vi "find_PrepLineObject_by_Koords.vi"(9 "Coords":T1, 10 "PrepLine\nobjects in":refnum<class "PrepLineObject.lvclass">[](array[class])) -> (0 "changed PrepLineObject":refnum<class "PrepLineObject.lvclass">, 1 "name of changed":string, 2 "changed switch array":bool[](array[boolean]), 3 "PrepLineObjectsOut":refnum<class "PrepLineObject.lvclass">[](array[class]))   [LabVIEW 2017]
doc: "According to coordinates the correct PrepLineObject is located by looking through the Array of all PrepLineObjects (stored in a queue). The output array has the same size as the array with the switch objects and shows (state = true) the location of the Object that that has been selected."
uses:
  <vilib>/Utility/miscctls.llb/LVPoint32TypeDef.ctl
  Classes/PrepLineObject/PrepLineObject.lvclass
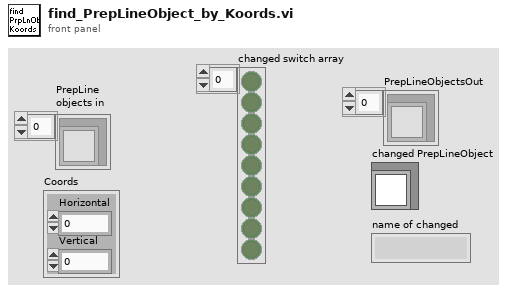
[diagram p1: front panel]
types:
  T1 = typedef "LVPoint32TypeDef.ctl" = cluster{"Horizontal":i32, "Vertical":i32}
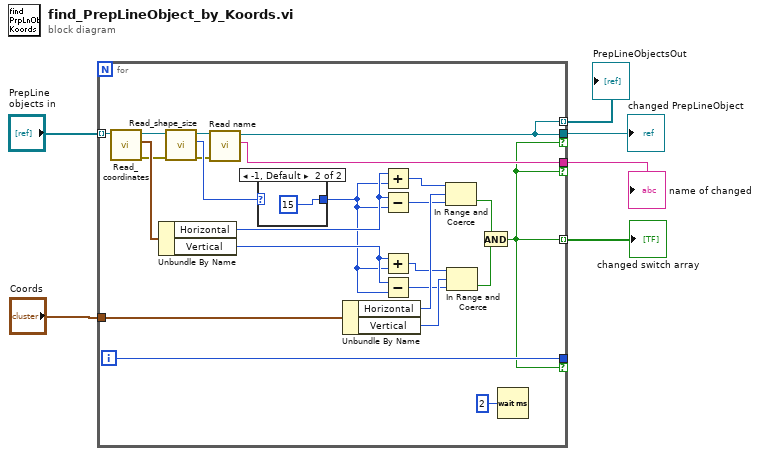
[diagram p0: block diagram]
diagram:
  n1 = for {
    tunnel: "PrepLine\nobjects in" -> [w30] mode=indexing
    tunnel: "Coords" -> [w28]
    tunnel: [w7] -> w5 mode=indexing
    tunnel: [w10] -> w4 if=w7
    tunnel: [w11] -> w3 if=w7
    tunnel: [w10] -> w1 mode=indexing
    tunnel: [w8] -> _ if=w7
    i -> [w8]
    n2 = call-dynamic "Read_coordinates.vi"("PrepLinePictureObjects in"=w30) -> ("PrepLinePictureObjects out"=w27:refnum<class "PrepLineObject.lvclass">, "Coords"=w29:T1, "error out"=w26:errorcluster)  [unwired: 7 in]
    n3 = Unbundle By Name(w29) -> ("Horizontal"=w24:i32, "Vertical"=w22:i32)
    n4 = call-dynamic "Read_shape_size.vi"("PrepLinePictureObjects in"=w27, "error in (no error)"=w26) -> ("PrepLinePictureObjects out"=w13:refnum<class "PrepLineObject.lvclass">, "shape type"=w15:i8, "error out"=w12:errorcluster)  [unwired: 6 in]
    n5 = call-dynamic "Read name.vi"("error in (no error)"=w12, "PrepLineObject in"=w13) -> ("name"=w11:string, "PrepLineObject out"=w10:refnum<class "PrepLineObject.lvclass">)  [unwired: 7 in, 1 out]
    n6 = case shown="-1, Default" w15 {
      selector: w15 -> [w31 _]
      tunnel: [w31 i8 15 ("shape type")] -> w14
      frame 0.. {
      }
      frame -1, Default {
      }
    }
    n7 = Unbundle By Name(w28) -> ("Horizontal"=w23:i32, "Vertical"=w25:i32)
    n8 = Add(x=w24, y=w14) -> (x+y=w21:i32)
    n9 = Subtract(x=w24, y=w14) -> (x-y=w20:i32)
    n10 = Add(x=w22, y=w14) -> (x+y=w19:i32)
    n11 = Subtract(x=w22, y=w14) -> (x-y=w18:i32)
    n12 = In Range and Coerce(upper limit=w21, x=w23, lower limit=w20) -> (In Range?=w17:bool)  [unwired: 1 out]
    n13 = In Range and Coerce(upper limit=w19, x=w25, lower limit=w18) -> (In Range?=w16:bool)  [unwired: 1 out]
    n14 = And(x=w17, y=w16) -> (x .and. y?=w7:bool)
    n15 = Wait (ms)(milliseconds to wait=u32 2) -> ()  [unwired: 1 out]
  }
  "changed switch array" <- w5
  "changed PrepLineObject" <- w4
  "name of changed" <- w3
  "PrepLineObjectsOut" <- w1
